vi "pulse Counter (SubVI).vi"(8 "error in (no error)":errorcluster, 11 "Waveform Graph":waveform(dbl)) -> (0 "error out":errorcluster, 3 "Numeric":i32)   [LabVIEW 2019]
uses:
  <vilib>/measure/mascope.llb/Cycle Average and RMS 1 chan.vi
  <vilib>/measure/NI_MAPro.lvlib
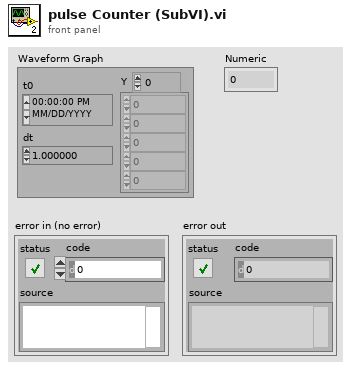
[diagram p1: front panel]
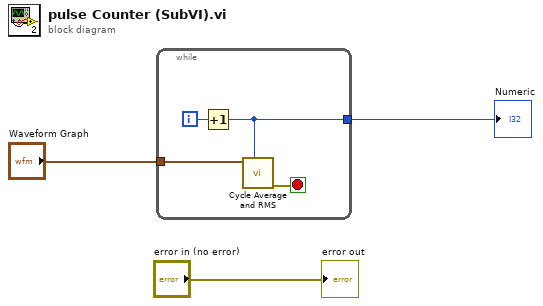
[diagram p0: block diagram]
diagram:
  n1 = while {
    tunnel: "Waveform Graph" -> [w7]
    tunnel: [w4] -> w3
    i -> [w6]
    stop <- w5 stop-if-true
    n2 = Increment(x=w6) -> (x+1=w4:i32)
    n3 = call-poly <vilib>:"Cycle Average and RMS.vi"("cycle number (1)"=w4, "signal in"=w7) -> ("error out"=w5:errorcluster)  [unwired: 6 in, 3 out]
  }
  "Numeric" <- w3
  "error out" <- "error in (no error)"
